vi "PassOrFail (SubVI).vi"(6 "String Res":string, 7 "index (row)":i32, 8 "error in (no error)":errorcluster, 9 "Data in":dbl format="%#_13g", 10 "Pass?Fail":bool, 11 "Table in":refnum<vi>) -> (0 "error out":errorcluster)   [LabVIEW 2017]
uses:
  <vilib>/Utility/miscctls.llb/LVRowAndColumnTypeDef.ctl
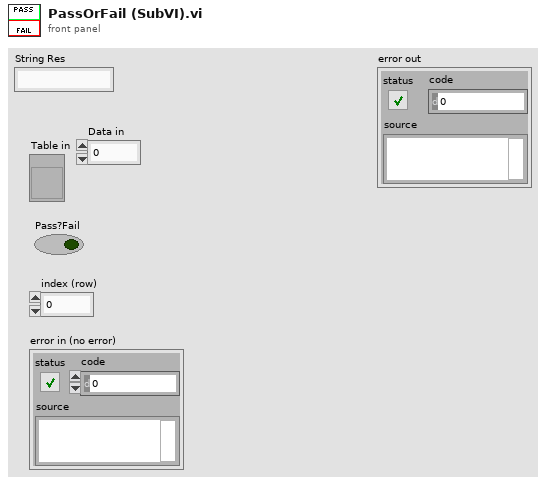
[diagram p1: front panel]
types:
  T1 = typedef "LVRowAndColumnTypeDef.ctl" = cluster{"Row":i32, "Column":i32}
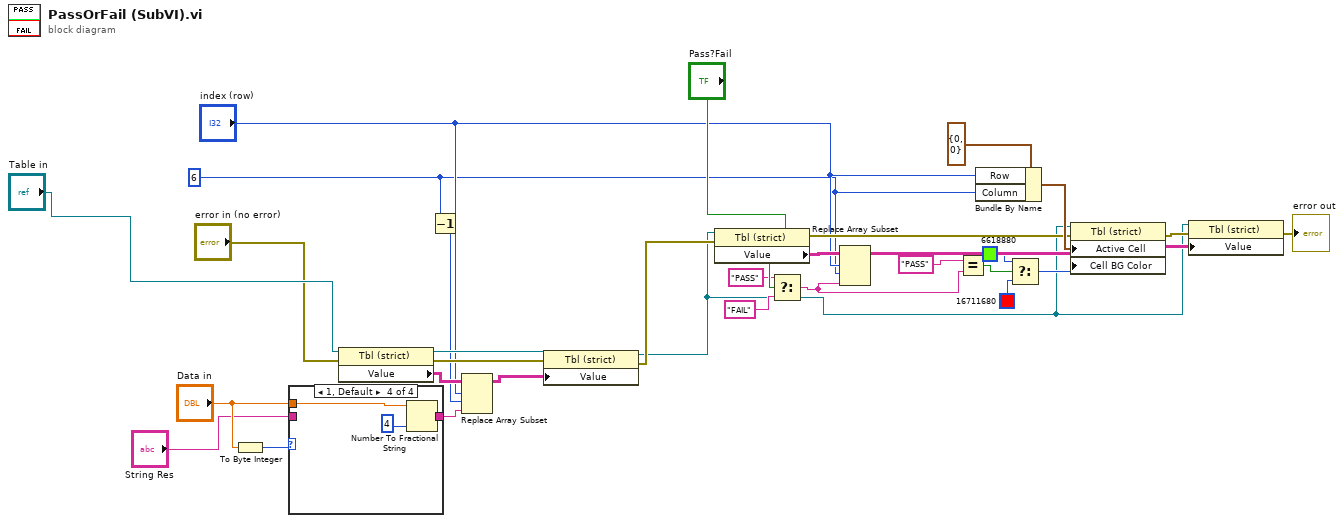
[diagram p0: block diagram]
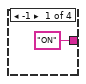
[diagram p2: hidden frame]
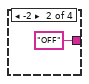
[diagram p3: hidden frame]
diagram:
  w5 = 6 ("disabled index (col)")
  n1 = To Byte Integer(number="Data in") -> (8bit integer=w2:i8)
  n2 = case shown="1, Default" w2 {
    tunnel: ["ON" "OFF" w34 w37] -> w7
    tunnel: "Data in" -> [_ _ _ w35]
    tunnel: "String Res" -> [_ _ w34 _]
    frame -1 {
    }
    frame -2 {
    }
    frame -3 {
    }
    frame 1, Default {
      n3 = Number To Fractional String(number=w35, precision (6)=i16 4) -> (F-format string=w37:string)  [unwired: 2 in]
    }
  }
  n4 = property class="Tbl (strict)"(reference="Table in", error in="error in (no error)") -> (reference out=w9:refnum<vi>, error out=w11:errorcluster, "Value"=w15:string[][])
  n5 = Decrement(x=w5) -> (x-1=w4:i32)
  n6 = Replace Array Subset(array=w15, new element=w7, index (row)="index (row)", index (col)=w4) -> (w14:string[][])
  n7 = property class="Tbl (strict)"(reference=w9, error in=w11, "Value"=w14) -> (reference out=w8:refnum<vi>, error out=w10:errorcluster)
  n8 = property class="Tbl (strict)"(reference=w8, error in=w10) -> (error out=w25:errorcluster, "Value"=w22:string[][])  [unwired: 1 out]
  n9 = Select(t="PASS" ("x"), s="Pass?Fail", f="FAIL" ("x")) -> (s? t:f=w28:string)
  n10 = Replace Array Subset(array=w22, new element=w28, index (row)="index (row)", index (col)=w5) -> (w23:string[][])
  n11 = Equal?(x="PASS", y=w28) -> (x = y?=w17:bool)
  n12 = Bundle By Name(cluster=T1 {"Row"=0, "Column"=0} ("Active Cell:Active Cell"), "Row"="index (row)", "Column"=w5) -> (w31:T1)
  n13 = Select(t=u32 6618880, s=w17, f=u32 16711680) -> (s? t:f=w21:u32)
  n14 = property class="Tbl (strict)"(reference=w8, error in=w25, "Active Cell"=w31, "Cell BG Color"=w21) -> (error out=w24:errorcluster)  [unwired: 1 out]
  n15 = property class="Tbl (strict)"(reference=w8, error in=w24, "Value"=w23) -> (error out=→"error out":errorcluster)  [unwired: 1 out]
